vi "RefInAndReset 2 PowerIndicator (uSMC).vi"(4 "Reset":bool, 5 "RefIn":bool) -> (1 "Power":u16)   [LabVIEW 2010, in "SignalWriterMH110203USBStepperMotor.lvclass"]
uses:
  SignalWriterMH110203USBStepperMotor.lvclass
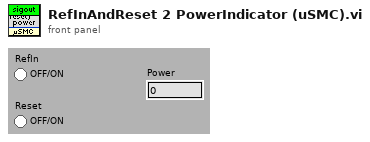
[diagram p1: front panel]
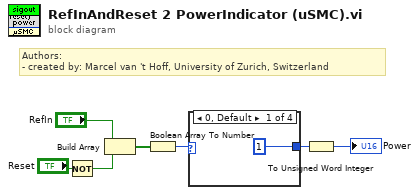
[diagram p0: block diagram]
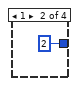
[diagram p2: hidden frame]
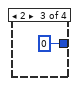
[diagram p3: hidden frame]
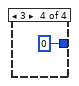
[diagram p4: hidden frame]
diagram:
  # "Authors: \n- created by: Marcel van 't Hoff, University of Zurich, Switzerland"
  n1 = Not(x="Reset") -> (.not. x?=w1:bool)
  n2 = Build Array("RefIn", w1) -> (w5:bool[])
  n3 = Boolean Array To Number(Boolean array=w5) -> (number=w4:u32)
  n4 = case shown="0, Default" w4 {
    tunnel: [1 2 0 0] -> w3
    frame 0, Default {
    }
    frame 1 {
    }
    frame 2 {
    }
    frame 3 {
    }
  }
  n5 = To Unsigned Word Integer(number=w3) -> (unsigned 16bit integer=→"Power":u16)
